vi "S4GUI Command Generator.vi"() -> (0 "error":errorcluster, 3 "command sent to S4ICS":string, 11 "response from S4ICS":string)   [LabVIEW 2018]
panel:
  in  "Status":bool
  out "Server":bool
  out "exec. ms":u32
  in  "Repeat":i32=1
  in  "test":bool
  in  "Address":string="localhost"
  in  "Port":u16=54165 min=1025 step=1
  in  "test stop":bool
  out "chart":dbl[](graph)
  out "Log":cluster{"sent":string, "rec":string}[](array[cluster])
  in  "stop":bool
  in  "commands":string(combo)="S4ICS" caption="Available S4GUI Commands"
  in  "Replace VALUE* by":dbl
  in  "ExecuteCmd":bool
  out "initial ms":u32
  # "S4GUI Command Simulator"
  # "(*) Position values can't use comma as decimal separator because\n     it is also used as command separator inside command message."
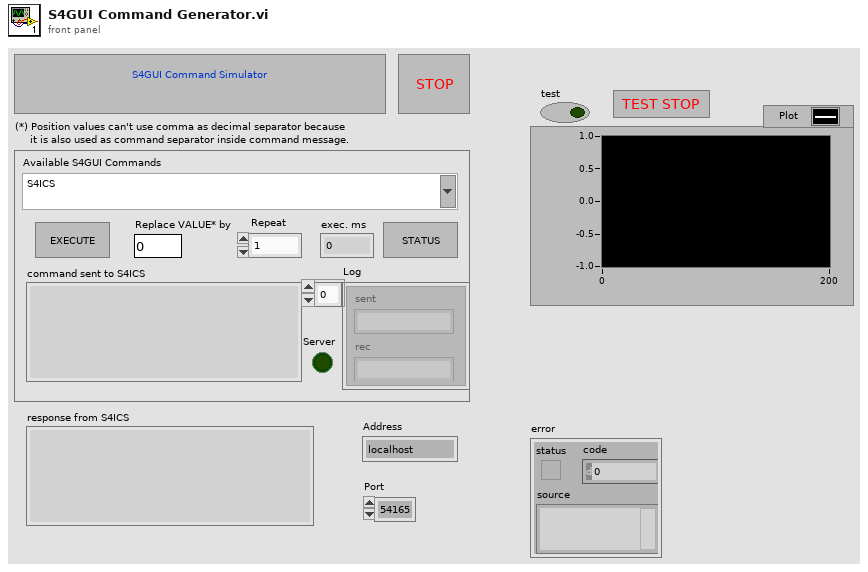
[diagram p1: front panel]
types:
  T1 = enum16{"Standard", "Buffered", "CRLF", "Immediate"}
  T2 = cluster{"result string":string, "result string":string}
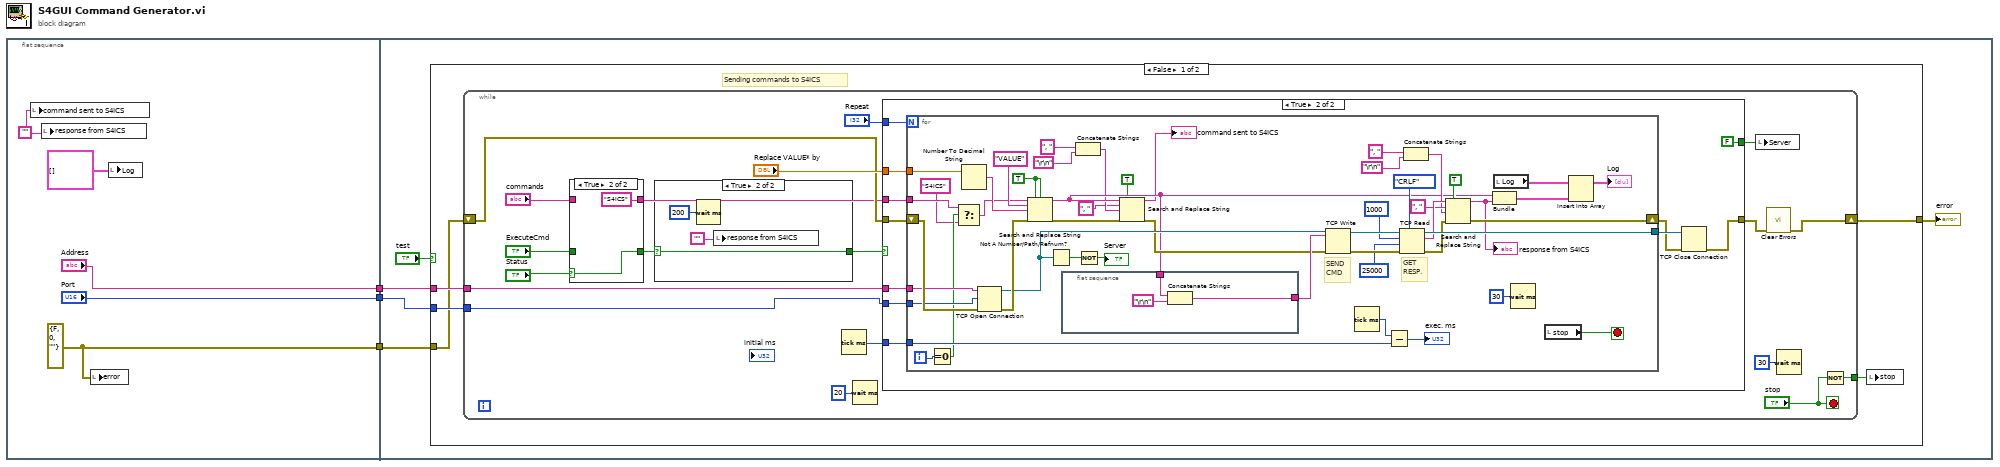
[diagram p0: block diagram]
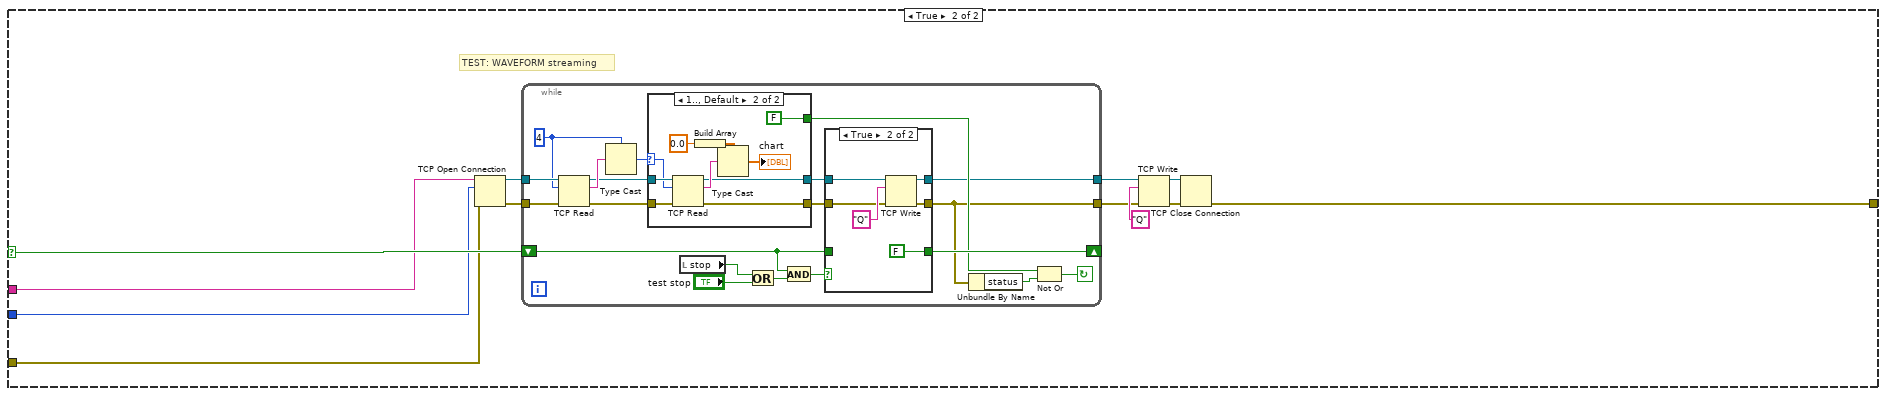
[diagram p5: hidden frame]
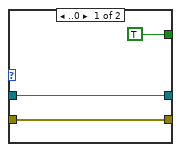
[diagram p7: hidden frame]
diagram:
  n1 = flat-sequence {
    tunnel: ["Address"] -> w3
    tunnel: ["Port"] -> w2
    tunnel: [w4] -> w1
    tunnel: w3 -> [w11]
    tunnel: w2 -> [w10]
    tunnel: w1 -> [w9]
    frame #0 {
      w5 = ""
      w4 = errorcluster {"status"=FALSE, "code"=0, "source"=""} ("error in")
      n2 = local write "command sent to S4ICS"(w5) -> ()
      n3 = local write "response from S4ICS"(w5) -> ()
      n4 = local write "error"(w4) -> ()
      n5 = local write "Log"(cluster{"sent":string, "rec":string}[] [] ("Log")) -> ()
    }
    frame #1 {
      n6 = case shown="False" "test" {
        selector: "test" -> [_ w115]
        tunnel: [w15 w121] -> w13
        tunnel: w11 -> [w18 w113]
        tunnel: w10 -> [w17 w112]
        tunnel: w9 -> [w16 w114]
        frame False {
          # "Sending commands to S4ICS"
          n7 = while {
            tunnel: w18 -> [w32]
            tunnel: w17 -> [w31]
            shift-right: [w29] -> w15
            shift-left: w16 -> [w35]
            tunnel: [w26] -> w14
            stop <- "stop" stop-if-true
            n8 = case shown="True" "Status" {
              selector: "Status" -> [_ w45]
              tunnel: "ExecuteCmd" -> [w42 _]
              tunnel: "commands" -> [w43 _]
              tunnel: [w43 "S4ICS"] -> w24
              tunnel: [w42 w45] -> w20
              frame False {
              }
              frame True {
              }
            }
            n9 = case shown="True" w20 {
              selector: w20 -> [w38 w41]
              tunnel: [w38 w41] -> w19
              frame False {
              }
              frame True {
                n10 = Wait (ms)(milliseconds to wait=u32 200) -> ()  [unwired: 1 out]
                n11 = local write "response from S4ICS"("") -> ()
              }
            }
            n12 = Tick Count (ms)() -> (millisecond timer value=w21:u32)
            n13 = Wait (ms)(milliseconds to wait=u32 20) -> ()  [unwired: 1 out]
            n14 = case shown="True" w19 {
              tunnel: "Replace VALUE* by" -> [_ w56]
              tunnel: w24 -> [_ w57]
              tunnel: w35 -> [w46 w55]
              tunnel: [w46 w48] -> w30
              tunnel: "Repeat" -> [_ w54]
              tunnel: [_ FALSE] -> w33
              tunnel: w32 -> [_ w52]
              tunnel: w31 -> [_ w51]
              tunnel: w21 -> [_ w47]
              frame False {
              }
              frame True {
                n15 = for {
                  N: w54 -> [_]
                  tunnel: w57 -> [w60]
                  tunnel: w56 -> [w106]
                  tunnel: [w104] -> w50
                  tunnel: w52 -> [w79]
                  tunnel: w51 -> [w78]
                  shift-right: [w105] -> w49
                  shift-left: w55 -> [w84]
                  tunnel: w47 -> [w63]
                  i -> [w61]
                  stop <- w85 stop-if-true
                  w100 = TRUE ("ignore case? (F)")
                  # "GET\nRESP."
                  # "SEND\nCMD"
                  n16 = Equal To 0?(x=w61) -> (x = 0?=w62:bool)
                  n17 = Select(t=w60, s=w62, f="S4ICS") -> (s? t:f=w59:string)
                  n18 = Number To Decimal String(number=w106) -> (decimal integer string=w103:string)  [unwired: 1 in]
                  n19 = TCP Open Connection(address=w79, remote port or service name=w78, error in (no error)=w84) -> (connection ID=w82:refnum<k5>, error out=w83:errorcluster)  [unwired: 2 out]
                  n20 = Search and Replace String(replace all?=w100, case sensitive?=w100, input string=w59, search string="VALUE", replace string=w103, error in=w83) -> (result string=w70:string, error out=w72:errorcluster)  [unwired: 2 in, 2 out]
                  n21 = Not A Number/Path/Refnum?(number/path/refnum=w82) -> (NaN/Path/Refnum?=w81:bool)
                  n22 = flat-sequence {
                    tunnel: [w108] -> w99
                    tunnel: w70 -> [w107]
                    frame #0 {
                      n23 = Concatenate Strings(w107, "\r\n") -> (w108:string)
                    }
                  }
                  n24 = Concatenate Strings(", " ("replace string (\"\")"), "\r\n") -> (w67:string)
                  n25 = Not(x=w81) -> (.not. x?=→"Server":bool)
                  n26 = Search and Replace String(replace all?=TRUE ("replace all? (F)"), input string=w70, search string=", ", replace string=w67, error in=w72) -> (result string=→"command sent to S4ICS":string, error out=w71:errorcluster)  [unwired: 3 in, 2 out]
                  n27 = TCP Write(connection ID=w82, data in=w99, error in (no error)=w71) -> (connection ID out=w102:refnum<k5>, error out=w101:errorcluster)  [unwired: 1 in, 1 out]
                  n28 = Tick Count (ms)() -> (millisecond timer value=w89:u32)
                  n29 = Subtract(x=w89, y=w63) -> (x-y=→"exec. ms":u32)
                  n30 = TCP Read(connection ID=w102, bytes to read=1000, error in (no error)=w101, 7:T1."CRLF" ("mode (standard)"), 9:25000 ("bytes to read")) -> (connection ID out=w104:refnum<k5>, data out=w93:string, error out=w88:errorcluster)
                  n31 = Concatenate Strings(", " ("replace string (\"\")"), "\r\n") -> (w74:string)
                  n32 = Search and Replace String(replace all?=TRUE ("replace all? (F)"), input string=w93, search string=", ", replace string=w74, error in=w88) -> (result string=w90:string, error out=w105:errorcluster)  [unwired: 3 in, 2 out]
                  "response from S4ICS" <- w90
                  n33 = Bundle("result string"=w70, "result string"=w90) -> (w97:T2)  [unwired: 1 in]
                  n34 = local read "Log"() -> (w95:cluster{"sent":string, "rec":string}[])
                  n35 = Wait (ms)(milliseconds to wait=u32 30) -> ()  [unwired: 1 out]
                  n36 = local read "stop"() -> (w85:bool)
                  n37 = Insert Into Array(array=w95, new element=w97) -> (→"Log":cluster{"sent":string, "rec":string}[])  [unwired: 1 in]
                }
                n38 = TCP Close Connection(connection ID=w50, error in (no error)=w49) -> (error out=w48:errorcluster)  [unwired: 1 in, 1 out]
              }
            }
            n39 = local write "Server"(w33) -> ()
            n40 = call <vilib>:"Clear Errors.vi"("error in (no error)"=w30) -> ("error out"=w29:errorcluster)  [unwired: 5 in, 1 out]
            n41 = Wait (ms)(milliseconds to wait=u32 30) -> ()  [unwired: 1 out]
            n42 = Not(x="stop") -> (.not. x?=w26:bool)
          }
          n43 = local write "stop"(w14) -> ()
        }
        frame True {
          # "TEST: WAVEFORM streaming"
          n44 = TCP Open Connection(address=w113, remote port or service name=w112, error in (no error)=w114) -> (connection ID=w111:refnum<k5>, error out=w110:errorcluster)  [unwired: 2 out]
          n45 = while {
            shift-left: w115 -> [w125]
            shift-right: [w135] -> _
            tunnel: w110 -> [w139]
            tunnel: w111 -> [w140]
            tunnel: [w130] -> w117
            tunnel: [w128] -> w119
            stop <- w126 continue-if-true
            w138 = 4
            n46 = TCP Read(connection ID=w140, bytes to read=w138, error in (no error)=w139) -> (connection ID out=w131:refnum<k5>, data out=w141:string, error out=w132:errorcluster)  [unwired: 2 out]
            n47 = Type Cast(type=w138, x=w141) -> (*(type *) &x=w137:i32)
            n48 = case shown="1.., Default" w137 {
              selector: w137 -> [_ w159]
              tunnel: w132 -> [w151 w162]
              tunnel: w131 -> [w153 w161]
              tunnel: [w153 w160] -> w129
              tunnel: [TRUE FALSE] -> w133
              tunnel: [w151 w157] -> w134
              frame ..0 {
              }
              frame 1.., Default {
                n49 = TCP Read(connection ID=w161, bytes to read=w159, error in (no error)=w162) -> (connection ID out=w160:refnum<k5>, data out=w163:string, error out=w157:errorcluster)  [unwired: 2 out]
                n50 = Build Array(0.0) -> (w155:dbl[])
                n51 = Type Cast(type=w155, x=w163) -> (*(type *) &x=→"chart":dbl[])
              }
            }
            n52 = local read "stop"() -> (w122:bool)
            n53 = Or(x=w122, y="test stop") -> (x .or. y?=w124:bool)
            n54 = And(x=w125, y=w124) -> (x .and. y?=w136:bool)
            n55 = case shown="True" w136 {
              tunnel: w125 -> [w143 _]
              tunnel: [w143 FALSE] -> w135
              tunnel: w129 -> [w142 w150]
              tunnel: w134 -> [w144 w147]
              tunnel: [w144 w146] -> w128
              tunnel: [w142 w145] -> w130
              frame False {
              }
              frame True {
                n56 = TCP Write(connection ID=w150, data in="Q", error in (no error)=w147) -> (connection ID out=w145:refnum<k5>, error out=w146:errorcluster)  [unwired: 2 out]
              }
            }
            n57 = Unbundle By Name(w128) -> ("status"=w127:bool)
            n58 = Not Or(1:w127, 2:w133) -> (0:w126:bool)
          }
          n59 = TCP Write(connection ID=w117, data in="Q", error in (no error)=w119) -> (connection ID out=w116:refnum<k5>, error out=w118:errorcluster)  [unwired: 2 out]
          n60 = TCP Close Connection(connection ID=w116, error in (no error)=w118) -> (error out=w121:errorcluster)  [unwired: 2 out]
        }
      }
      "error" <- w13
    }
  }
